vi "SetButtonDefinitionFile.vi"(8 "Error In":errorcluster, 10 "ButtonDefinitionFile":string, 11 "reference in":refnum<class "TemplateGUI.lvclass">) -> (0 "Error Out":errorcluster, 3 "reference out":refnum<class "TemplateGUI.lvclass">)   [LabVIEW 2021]
uses:
  TemplateGUI.lvclass/TemplateGUI.ctl
  TemplateGUI.lvclass
  VerticalButtonBar/ButtonCollection/ButtonCollection.lvclass
  .Externals/Library_TSFramework_ApplicationArchitecture/Application/Application.lvclass
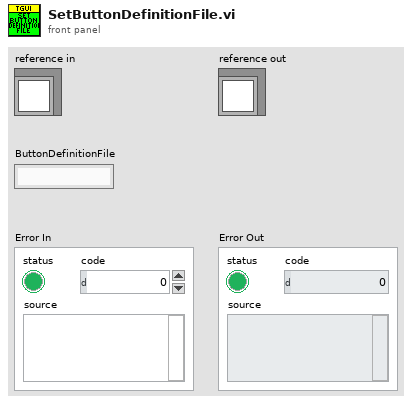
[diagram p1: front panel]
types:
  T1 = typedef "TemplateGUI.lvclass/ObjectAttributes.ctl" = cluster{"Interfaces":cluster{"Dummys":refnum<class>}, "Locals":cluster{"Dummy":bool}, "Persistent":cluster{"Dummy":bool}}
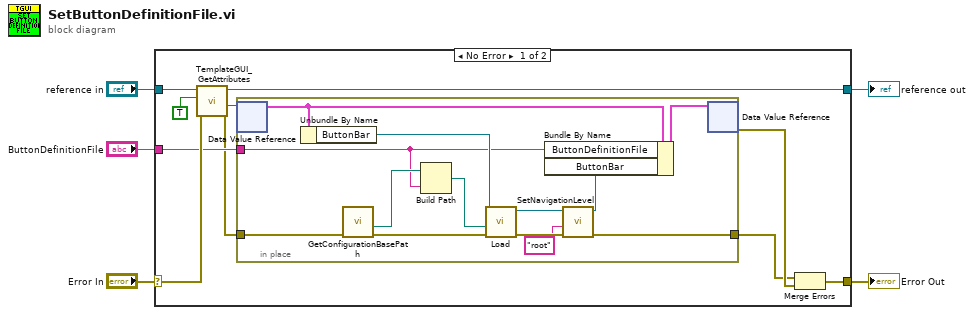
[diagram p0: block diagram]
diagram:
  n1 = case shown="No Error" "Error In" {
    selector: "Error In" -> [w15 w30]
    tunnel: [w13 w30] -> w4
    tunnel: [w11 w29] -> w2
    tunnel: "reference in" -> [w12 w29]
    tunnel: "ButtonDefinitionFile" -> [w8 _]
    frame No Error {
      n2 = call "TemplateGUI_GetAttributes.vi"("error in (no error)"=w15, "OnlyGetDvrReference(False)"=TRUE, "reference in"=w12) -> ("error out"=w7:errorcluster, "DataRef"=w9:refnum<data-value>, "reference out"=w11:refnum<class "TemplateGUI.lvclass">)  [unwired: 5 in, 1 out]
      n3 = in-place {
        in-place-border: w8 -> [w17]
        in-place-border: w7 -> [w20]
        in-place-border: [w24] -> w6
        n4 = in-place-dvr #1(w9) -> (w26:T1)  [unwired: 1 out]
        n5 = Unbundle By Name(w26) -> ("ButtonBar"=w25:refnum<class "ButtonCollection.lvclass">)
        n6 = call "GetConfigurationBasePath.vi"("Error In"=w20) -> ("Error Out"=w19:errorcluster, "BasePath"=w18:path)  [unwired: 9 in]
        n7 = Build Path(base path=w18, name or relative path=w17) -> (appended path=w16:path)
        n8 = call "Load.vi"("ErrorIn"=w19, "Path"=w16, "ObjectIn"=w25) -> ("ErrorOut"=w27:errorcluster, "ObjectOut"=w23:refnum<class "ButtonCollection.lvclass">)  [unwired: 7 in]
        n9 = call-dynamic "SetNavigationLevel.vi"("ErrorIn"=w27, "NavigationName"="root", "ObjectIn"=w23) -> ("ErrorOut"=w24:errorcluster, "ObjectOut"=w21:refnum<class "ButtonCollection.lvclass">)  [unwired: 7 in]
        n10 = Bundle By Name(cluster=w26, "ButtonDefinitionFile"=w17, "ButtonBar"=w21) -> (w28:T1)
        n11 = in-place-dvr #1(w28) -> (w14:errorcluster)  [unwired: 1 out]
      }
      n12 = Merge Errors(w6, w14) -> (w13:errorcluster)
    }
    frame Error {
    }
  }
  "Error Out" <- w4
  "reference out" <- w2
